vi "Cannon Global Data.vi"() -> ()   [LabVIEW 2013]
uses:
  <vilib>/Rock Robotics/WPI/Solenoid/WPI_SolenoidValue.ctl
panel:
  in  "Cannon Global Data":T2
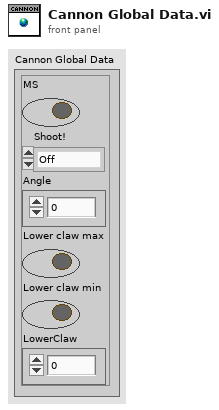
[diagram p1: front panel]
types:
  T1 = typedef "WPI_SolenoidValue.ctl" = enum16{"Off", "On", "Forward", "Reverse"}
  T2 = cluster{"MS":bool, "Shoot!":T1, "Angle":dbl, "Lower claw max":bool, "Lower claw min":bool, "LowerClaw":dbl}
diagram:
